vi "Fc_Get_TRACEDATA.vi"(6 "Start+timeout?":bool, 8 "error in (no error)":errorcluster, 11 "Class TCP in":T1) -> (0 "error out":errorcluster, 3 "Class TCP out":T1)   [LabVIEW 2021]
doc: "This function calls the microcontroller to obtain the signal data and stores them at the time of the request, into the \"Signals_value_Array\" variable."
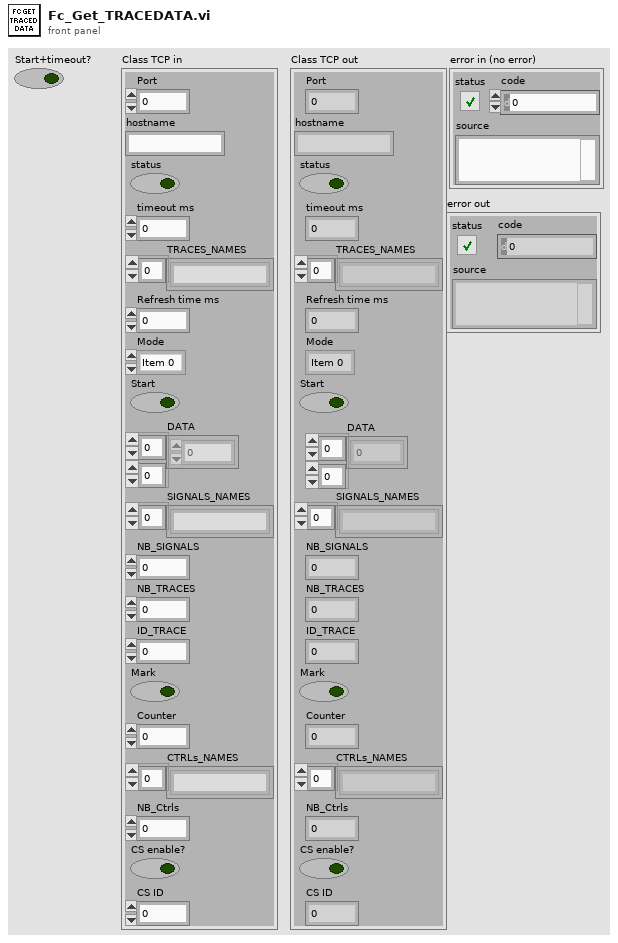
[diagram p1: front panel]
types:
  T1 = cluster{"Port":i32, "hostname":string, "status":bool, "timeout ms":i32, "TRACES_NAMES":string[], "Refresh time ms":i32, "Mode":enum32{"Item 0", "Item 1"}, "Start":bool, "DATA":sgl[][], "SIGNALS_NAMES":string[], "NB_SIGNALS":i32, "NB_TRACES":i32, "ID_TRACE":i32, "Mark":bool, "Counter":i32, "CTRLs_NAMES":string[], "NB_Ctrls":i32, "CS enable?":bool, "CS ID":i32}
  T2 = cluster{"TRACE_SIZE":i32, "CS_ID":i32, "TRACE ID":i32, "CMD":i32, "DATA(M)":i32}
  T3 = cluster{"timeout ms":i32, "remote port":u16, "Address":string}
  T4 = cluster{"SIZE":i32, " TRACE DATA":sgl[], "TRACE_SIZE":i32, "NB_TRACES":i32, "NB_TRACED_SIGNALS":i32, "NAMES TRACED SIGNALS":string[], "NAMES TRACES":string[], "CS STATUS":i32, "NB_CSs":i32, "NAMES CSs":string[], "DATA (M)":sgl[], "CMD":i32}
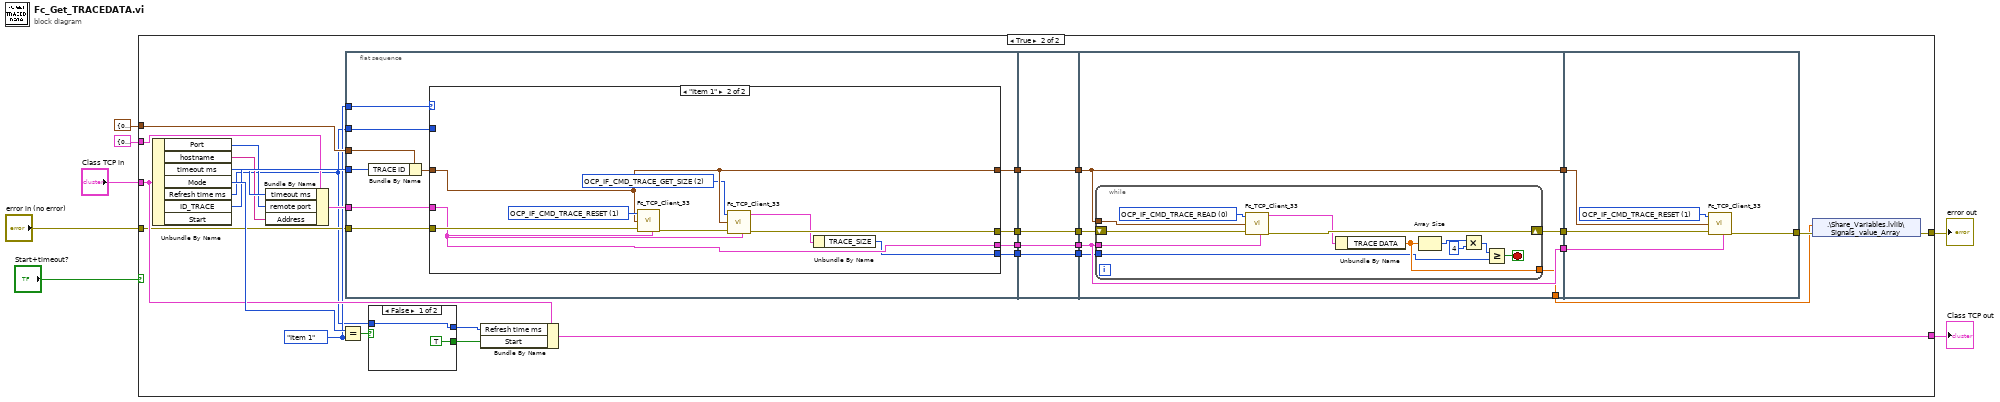
[diagram p0: block diagram]
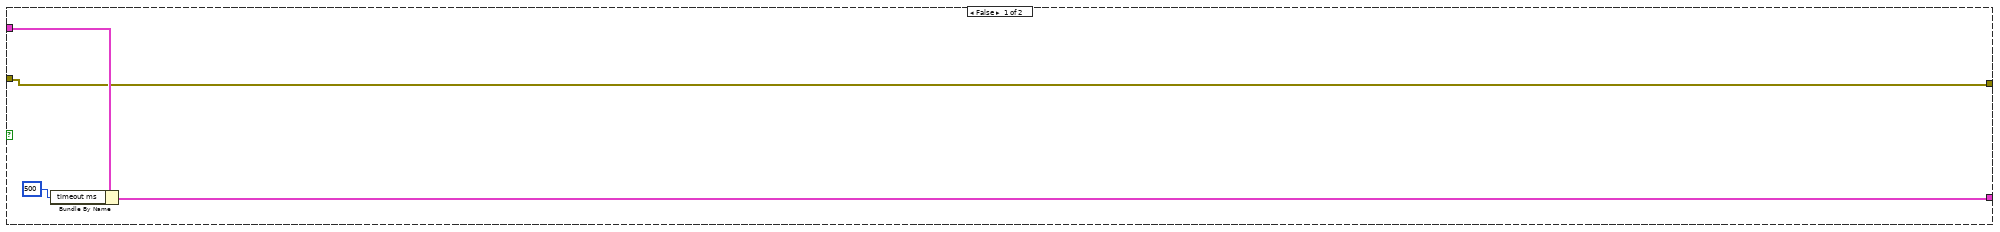
[diagram p2: hidden frame]
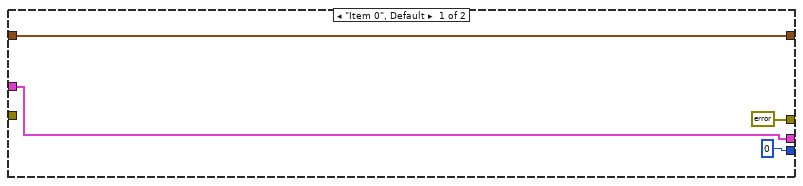
[diagram p3: hidden frame]
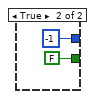
[diagram p4: hidden frame]
diagram:
  n1 = case shown="True" "Start+timeout?" {
    tunnel: "Class TCP in" -> [w11 w25]
    tunnel: [w10 w36] -> w5
    tunnel: T2 {"TRACE_SIZE"=0, "CS_ID"=0, "TRACE ID"=0, "CMD"=0, "DATA(M)"=0} ("Input Cluster") -> [_ w27]
    tunnel: T3 {"timeout ms"=0, "remote port"=0, "Address"=""} ("Comunication Cluster") -> [_ w26]
    tunnel: "error in (no error)" -> [w8 w23]
    tunnel: [w8 w22] -> w1
    frame False {
      n2 = Bundle By Name(cluster=w11, "timeout ms"=500) -> (w10:T1)
    }
    frame True {
      w24 = enum32{"Item 0", "Item 1"}."Item 1" ("Mode")
      n3 = Unbundle By Name(w25) -> ("Port"=w31:i32, "hostname"=w30:string, "timeout ms"=w32:i32, "Mode"=w41:enum32{"Item 0", "Item 1"}, "Refresh time ms"=w12:i32, "ID_TRACE"=w38:i32)  [unwired: 1 out]
      n4 = Bundle By Name(cluster=w26, "timeout ms"=w32, "remote port"=w31, "Address"=w30) -> (w29:T3)
      n5 = Equal?(x=w41, y=w24) -> (x = y?=w40:bool)
      n6 = flat-sequence {
        tunnel: w29 -> [w50]
        tunnel: w27 -> [w46]
        tunnel: w38 -> [w52]
        tunnel: [w51] -> w20
        tunnel: [w49] -> w18
        tunnel: [w48] -> w16
        tunnel: w24 -> [w47]
        tunnel: w23 -> [w44]
        tunnel: [w43] -> w14
        tunnel: w12 -> [w42]
        tunnel: w20 -> [w69]
        tunnel: [w69] -> w19
        tunnel: w18 -> [w68]
        tunnel: [w68] -> w17
        tunnel: w16 -> [w67]
        tunnel: [w67] -> w15
        tunnel: w14 -> [w66]
        tunnel: [w66] -> w13
        tunnel: [w75] -> w37
        tunnel: [w72] -> w34
        tunnel: [w74] -> w33
        tunnel: w19 -> [w72]
        tunnel: w17 -> [w74]
        tunnel: w15 -> [w73]
        tunnel: [w71] -> w21
        tunnel: w13 -> [w70]
        tunnel: w37 -> [w92]
        tunnel: w34 -> [w91]
        tunnel: w33 -> [w90]
        tunnel: [w88] -> w28
        frame #0 {
          n7 = Bundle By Name(cluster=w46, "TRACE ID"=w52) -> (w45:T2)
          n8 = case shown="\"Item 1\"" w47 {
            tunnel: [w54 w63] -> w51
            tunnel: w50 -> [w55 w61]
            tunnel: [w55 w61] -> w49
            tunnel: [errorcluster {"status"=FALSE, "code"=0, "source"=""} ("error out") w60] -> w48
            tunnel: w45 -> [w54 w63]
            tunnel: w44 -> [_ w64]
            tunnel: [0 ("TRACE_SIZE") w57] -> w43
            tunnel: w42 -> [_ _]
            frame "Item 0", Default {
            }
            frame "Item 1" {
              w59 = 2 items=["OCP_IF_CMD_TRACE_READ", "OCP_IF_CMD_TRACE_RESET", "OCP_IF_CMD_TRACE_GET_SIZE", "OCP_IF_CMD_TRACE_SET_SIZE", "OCP_IF_CMD_TRACE_GET_NUMBER_SIGNALS", "OCP_IF_CMD_TRACE_GET_SIGNALS_NAMES", "OCP_IF_CMD_TRACE_GET_NUMBER_TRACES", "OCP_IF_CMD_TRACE_GET_TRACES_NAMES", "OCP_IF_CMD_TRACE_GET_ADDRESS", "OCP_IF_CMD_CS_STATUS", "OCP_IF_CMD_CS_ENABLE", "OCP_IF_CMD_CS_DISABLE", "OCP_IF_CMD_CS_CONTROLLER_IF", "OCP_IF_CMD_CS_HARDWARE_IF", "OCP_IF_CMD_CS_GET_NUMBER_CONTROLLERS", "OCP_IF_CMD_CS_GET_CONTROLLERS_NAMES", "OCP_IF_CMD_PLATFORM_ID", "OCP_IF_CMD_PLATFORM_IF", "OCP_IF_CMD_OPIL_UPDATE_MEASUREMENTS", "OCP_IF_CMD_OPIL_UPDATE_SIM_DATA", "OCP_IF_CMD_OPIL_RUN_CONTROL", "OCP_IF_CMD_OPIL_INITIALIZE_CONTROL", "OCP_IF_CMD_OPIL_GET_CONTROL", "OCP_IF_CMD_OPIL_GET_CONTROLLER_DATA", "OCP_IF_CMD_END"] ("CMD")
              w65 = 1 items=["OCP_IF_CMD_TRACE_READ", "OCP_IF_CMD_TRACE_RESET", "OCP_IF_CMD_TRACE_GET_SIZE", "OCP_IF_CMD_TRACE_SET_SIZE", "OCP_IF_CMD_TRACE_GET_NUMBER_SIGNALS", "OCP_IF_CMD_TRACE_GET_SIGNALS_NAMES", "OCP_IF_CMD_TRACE_GET_NUMBER_TRACES", "OCP_IF_CMD_TRACE_GET_TRACES_NAMES", "OCP_IF_CMD_TRACE_GET_ADDRESS", "OCP_IF_CMD_CS_STATUS", "OCP_IF_CMD_CS_ENABLE", "OCP_IF_CMD_CS_DISABLE", "OCP_IF_CMD_CS_CONTROLLER_IF", "OCP_IF_CMD_CS_HARDWARE_IF", "OCP_IF_CMD_CS_GET_NUMBER_CONTROLLERS", "OCP_IF_CMD_CS_GET_CONTROLLERS_NAMES", "OCP_IF_CMD_PLATFORM_ID", "OCP_IF_CMD_PLATFORM_IF", "OCP_IF_CMD_OPIL_UPDATE_MEASUREMENTS", "OCP_IF_CMD_OPIL_UPDATE_SIM_DATA", "OCP_IF_CMD_OPIL_RUN_CONTROL", "OCP_IF_CMD_OPIL_INITIALIZE_CONTROL", "OCP_IF_CMD_OPIL_GET_CONTROL", "OCP_IF_CMD_OPIL_GET_CONTROLLER_DATA", "OCP_IF_CMD_END"] ("CMD")
              n9 = call "Fc_TCP_Client_33.vi"("CMD"=w65, "Input Cluster"=w63, "error in (no error)"=w64, "Comunication Cluster"=w61) -> ("error out"=w62:errorcluster)  [unwired: 4 in, 2 out]
              n10 = call "Fc_TCP_Client_33.vi"("CMD"=w59, "Input Cluster"=w63, "error in (no error)"=w62, "Comunication Cluster"=w61) -> ("Output cluster"=w58:T4, "error out"=w60:errorcluster)  [unwired: 4 in, 1 out]
              n11 = Unbundle By Name(w58) -> ("TRACE_SIZE"=w57:i32)
            }
          }
        }
        frame #1 {
        }
        frame #2 {
          n12 = while {
            tunnel: w74 -> [w85]
            tunnel: w72 -> [w83]
            tunnel: [w81] -> w71
            shift-right: [w87] -> w75
            shift-left: w73 -> [w84]
            tunnel: w70 -> [w77]
            stop <- w76 stop-if-true
            w86 = 0 items=["OCP_IF_CMD_TRACE_READ", "OCP_IF_CMD_TRACE_RESET", "OCP_IF_CMD_TRACE_GET_SIZE", "OCP_IF_CMD_TRACE_SET_SIZE", "OCP_IF_CMD_TRACE_GET_NUMBER_SIGNALS", "OCP_IF_CMD_TRACE_GET_SIGNALS_NAMES", "OCP_IF_CMD_TRACE_GET_NUMBER_TRACES", "OCP_IF_CMD_TRACE_GET_TRACES_NAMES", "OCP_IF_CMD_TRACE_GET_ADDRESS", "OCP_IF_CMD_CS_STATUS", "OCP_IF_CMD_CS_ENABLE", "OCP_IF_CMD_CS_DISABLE", "OCP_IF_CMD_CS_CONTROLLER_IF", "OCP_IF_CMD_CS_HARDWARE_IF", "OCP_IF_CMD_CS_GET_NUMBER_CONTROLLERS", "OCP_IF_CMD_CS_GET_CONTROLLERS_NAMES", "OCP_IF_CMD_PLATFORM_ID", "OCP_IF_CMD_PLATFORM_IF", "OCP_IF_CMD_OPIL_UPDATE_MEASUREMENTS", "OCP_IF_CMD_OPIL_UPDATE_SIM_DATA", "OCP_IF_CMD_OPIL_RUN_CONTROL", "OCP_IF_CMD_OPIL_INITIALIZE_CONTROL", "OCP_IF_CMD_OPIL_GET_CONTROL", "OCP_IF_CMD_OPIL_GET_CONTROLLER_DATA", "OCP_IF_CMD_END"] ("CMD")
            n13 = call "Fc_TCP_Client_33.vi"("CMD"=w86, "Input Cluster"=w83, "error in (no error)"=w84, "Comunication Cluster"=w85) -> ("Output cluster"=w82:T4, "error out"=w87:errorcluster)  [unwired: 4 in, 1 out]
            n14 = Unbundle By Name(w82) -> ("TRACE DATA"=w81:sgl[])
            n15 = Array Size(array=w81) -> (size(s)=w80:i32)
            n16 = Multiply(x=w80, y=4) -> (x*y=w78:i32)
            n17 = Greater Or Equal?(x=w78, y=w77) -> (x >= y?=w76:bool)
          }
        }
        frame #3 {
          w89 = 1 items=["OCP_IF_CMD_TRACE_READ", "OCP_IF_CMD_TRACE_RESET", "OCP_IF_CMD_TRACE_GET_SIZE", "OCP_IF_CMD_TRACE_SET_SIZE", "OCP_IF_CMD_TRACE_GET_NUMBER_SIGNALS", "OCP_IF_CMD_TRACE_GET_SIGNALS_NAMES", "OCP_IF_CMD_TRACE_GET_NUMBER_TRACES", "OCP_IF_CMD_TRACE_GET_TRACES_NAMES", "OCP_IF_CMD_TRACE_GET_ADDRESS", "OCP_IF_CMD_CS_STATUS", "OCP_IF_CMD_CS_ENABLE", "OCP_IF_CMD_CS_DISABLE", "OCP_IF_CMD_CS_CONTROLLER_IF", "OCP_IF_CMD_CS_HARDWARE_IF", "OCP_IF_CMD_CS_GET_NUMBER_CONTROLLERS", "OCP_IF_CMD_CS_GET_CONTROLLERS_NAMES", "OCP_IF_CMD_PLATFORM_ID", "OCP_IF_CMD_PLATFORM_IF", "OCP_IF_CMD_OPIL_UPDATE_MEASUREMENTS", "OCP_IF_CMD_OPIL_UPDATE_SIM_DATA", "OCP_IF_CMD_OPIL_RUN_CONTROL", "OCP_IF_CMD_OPIL_INITIALIZE_CONTROL", "OCP_IF_CMD_OPIL_GET_CONTROL", "OCP_IF_CMD_OPIL_GET_CONTROLLER_DATA", "OCP_IF_CMD_END"] ("CMD")
          n18 = call "Fc_TCP_Client_33.vi"("CMD"=w89, "Input Cluster"=w91, "error in (no error)"=w92, "Comunication Cluster"=w90) -> ("error out"=w88:errorcluster)  [unwired: 4 in, 2 out]
        }
      }
      n19 = case shown="False" w40 {
        tunnel: [TRUE FALSE] -> w39
        tunnel: [w93 i8 -1 ("t")] -> w35
        tunnel: w12 -> [w93 _]
        frame False {
        }
        frame True {
        }
      }
      n20 = Bundle By Name(cluster=w25, "Refresh time ms"=w35, "Start"=w39) -> (w36:T1)
      n21 = shared-variable ".\\Share_Variables.lvlib\\Signals_value_Array"(w21, error in=w28) -> (error out=w22:errorcluster)
    }
  }
  "Class TCP out" <- w5
  "error out" <- w1
